vi "Get control names IQ PID.vi"() -> (3 "Names":string[](array[string]))   [LabVIEW 2018]
uses:
  Scope/controls/All FP controls.ctl
  FPGA/PID/PID control enabled type.ctl
  <vilib>/Analysis/4window.llb/windowTd.ctl
  Scope/controls/power_spectrum_unit.ctl
  FPGA/DataMode.ctl
  Scope5782/Scope/controls/5782_trigger_type.ctl
  Scope/controls/Output scale.ctl
  Scope/controls/host_transfer_speed.ctl
  FPGA/cavity model/Piezo setting.ctl
  <vilib>/Analysis/NI_AALPro.lvlib
panel:
  in  "All FP controls":T1
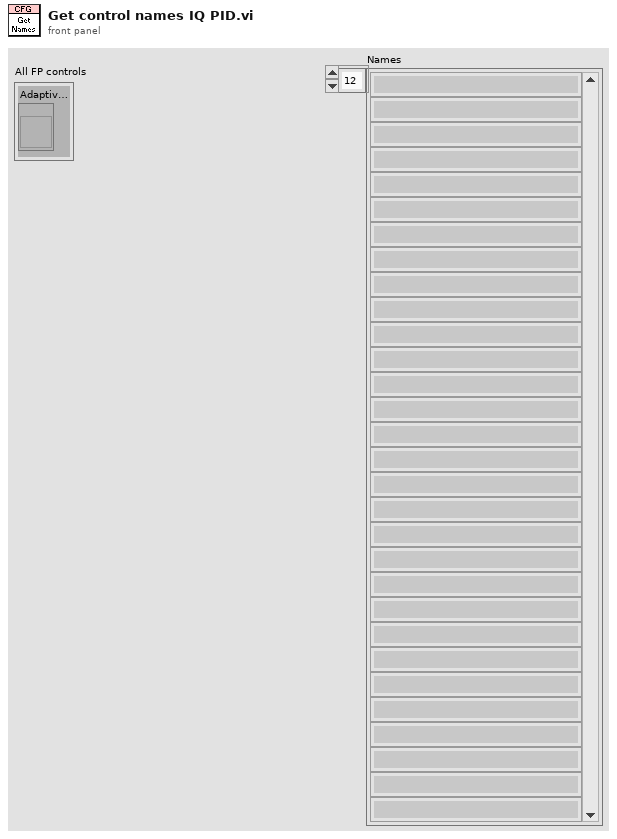
[diagram p1: front panel]
types:
  T1 = typedef "All FP controls.ctl" = cluster{"Adaptive FF enabled":refnum<vi>, "LP filter cutoff fequency [MHz]":refnum<vi>, "Adaptation factor [0-1]":refnum<vi>, "Samples to skip":refnum<vi>, "ch1 DC offset":refnum<vi>, "ch0 DC offset":refnum<vi>, "ch1 DC offset 2":refnum<vi>, "ch0 DC offset 2":refnum<vi>, "ch3 DC offset":refnum<vi>, "ch2 DC offset":refnum<vi>, "Feedback Q":refnum<vi>, "Ki*T Q":refnum<vi>, "Kd/T  Q":refnum<vi>, "Kp Q":refnum<vi>, "Acquire samples":refnum<vi>, "Trigger delay":refnum<vi>, "Feedback delay":refnum<vi>, "Kp AM":refnum<vi>, "Kd/T AM":refnum<vi>, "Ki*T AM":refnum<vi>, "Feedback I":refnum<vi>, "#bins":refnum<vi>, "Window":refnum<vi>, "Unit":refnum<vi>, "Input delay 5761":refnum<vi>, "Input delay 5785":refnum<vi>, "S":refnum<vi>, "K1":refnum<vi>, "Q1":refnum<vi>, "R1":refnum<vi>, "w12":refnum<vi>, "Cavity model":refnum<vi>, "w1":refnum<vi>, "Mode":refnum<vi>, "Trigger":refnum<vi>, "Output mixer fequency [MHz]":refnum<vi>, "Output delay":refnum<vi>, "Mixer freq [MHz]":refnum<vi>, "Triggered":refnum<vi>, "Continuous":refnum<vi>, "Output scale":refnum<vi>, "Host scale":refnum<vi>, "Input scale":refnum<vi>, "IIR filter cutoff fequency [MHz]":refnum<vi>, "Host scale 5761":refnum<vi>, "Virtual cavity":refnum<vi>, "Input scale 5761":refnum<vi>, "Tranfer speed":refnum<vi>, "Count to skip 5782, stage 1":refnum<vi>, "Count to skip 5761, stage 1":refnum<vi>, "K2":refnum<vi>, "w2":refnum<vi>, "K3":refnum<vi>, "Q3":refnum<vi>, "Q2":refnum<vi>, "w3":refnum<vi>, "w0":refnum<vi>, "Piezo":refnum<vi>, "Measure Tau at Time":refnum<vi>, "Tau set":refnum<vi>, "Count to skip 5761, stage 2":refnum<vi>, "Count to skip 5761, stage 3":refnum<vi>, "Count to skip 5782, stage 2":refnum<vi>, "Count to skip 5782, stage 3":refnum<vi>}
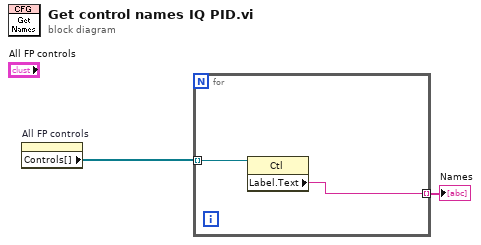
[diagram p0: block diagram]
diagram:
  n1 = property on="All FP controls" class="Clust (strict)"() -> ("Controls[]"=w2:refnum<vi>[])  [unwired: 2 in, 2 out]
  n2 = for {
    tunnel: w2 -> [w4] mode=indexing
    tunnel: [w3] -> w1 mode=indexing
    n3 = property class="Ctl"(reference=w4) -> ("Label.Text"=w3:string)  [unwired: 1 in, 2 out]
  }
  "Names" <- w1
